vi "network_test_usrp.vi"() -> ()   [LabVIEW 2021]
uses:
  FPGA/reciver params.ctl
  Host/SubVIs/Start Trigger.ctl
  <instrlib>/niUsrpRio/Config/v1/Host/Public/niUsrpRio Session.ctl
  <instrlib>/_niInstr/Register Bus/v0/Host/Public/Register Bus Session.ctl
  <instrlib>/_niInstr/Register Bus/v0/Host/Private/Session Data.ctl
  <instrlib>/niUsrpRio/Config/v1/Host/Private/DB Queue Reference.ctl
  <instrlib>/niUsrpRio/Config/v1/Host/Private/Daughterboard Data.ctl
  <instrlib>/niUsrpRio/Config/v1/Host/Private/ATR state data.ctl
  <instrlib>/niUsrpRio/Config/v1/Host/Private/Antenna Configuration.ctl
  <instrlib>/niUsrpRio/Config/v1/Host/Private/CPLD Power Mode.ctl
  <instrlib>/niUsrpRio/Config/v1/Host/Public/EEPROM Header.ctl
  <instrlib>/niUsrpRio/Config/v1/Host/Public/EEPROM Device Data Header.ctl
  <instrlib>/niUsrpRio/Config/v1/Host/Public/EEPROM Characterization Header.ctl
  <instrlib>/niUsrpRio/Config/v1/Host/Public/Characterization Data.ctl
  <instrlib>/niUsrpRio/Config/v1/Host/Public/IQ Imbalance.ctl
  Host/SubVIs/Streaming Xvcr FPGA Ref.ctl
  <vilib>/userDefined/Silver/nirio_resource_slv.ctl
  Host/SubVIs/Initiate and Fetch (Multi).vi
  Host/SubVIs/Initiate and Fetch Time (Multi).vi
  <vilib>/Utility/error.llb/Error Cluster From Error Code.vi
  <vilib>/rvi/errors/niLvFpgaAdjustHostInterfaceError.vi
  Host/SubVIs/Initiate and Trigger.vi
  Host/SubVIs/Fetch Rx Data.vi
  Host/SubVIs/Fetch Rx Data (CDB WDT).vi
  Host/SubVIs/Check Aurora Link.vi
  Host/SubVIs/Check Stream Status.vi
  <vilib>/rvi/interface/nirviReadWriteControl/nirviReadWriteControl.xnode
  <vilib>/rvi/interface/nirviMethod/nirviMethod.xnode
  NiFpgaLv.dll
  <vilib>/rvi/interface/Simulation/niFpgaSimulationCallBeginRW.vi
  <vilib>/FPGAPlugInAG/Dynamic/niLvFpga_ReadFifo_Dynamic.vi
  <vilib>/rvi/errors/niLvFpgaMergeErrorWithErrorCode.vi
  <instrlib>/_niInstr/Register Bus/v0/Host/niInstr Register Bus v0 Host.lvlib
  <instrlib>/niUsrpRio/Config/v1/Host/niUsrpRio Config v1 Host.lvlib
  <vilib>/FPGAPlugInAG/Dynamic/niLvFpga_StopFifo_Dynamic.vi
  <vilib>/FPGAPlugInAG/Dynamic/niLvFpga_StartFifo_Dynamic.vi
panel:
  out "Ip - controler":string
  out "oders obay":dbl
  out "error out":errorcluster
  out "packege sent":u64
  out "state":T1(ring)
  out "data out 2":string
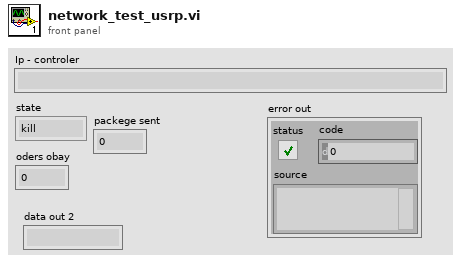
[diagram p1: front panel]
types:
  T1 = enum16{"kill", "turn off", "wait", "run", "turn on"}
  T2 = typedef "reciver params.ctl" = cluster{"min PW (fft cycels)":u16, "max PW (fft cycels)":u16, "max gap (fft cycels)":u8, "detection bar (liniar amp)":fxp<+,64,63>, "peak detect":bool}
  T3 = typedef "Start Trigger.ctl" = enum8{"Software", "Digital Edge", "Rx Start Trigger", "Tx Start Trigger", "Immediate", "Future Time Event"}
  T4 = typedef "niUsrpRio Config v1 Host.lvlib/niUsrpRio Session.ctl" = cluster{"FPGA Interface":refnum<k20>, "RIO Interface Number":u32, "Data Clock Rate":u32, "FPGA Data Clock Rate":u32, "Global Settings Register Bus":T5, "Radio 0 Settings Register Bus":T5, "Radio 1 Settings Register Bus":T5, "Radio Settings Bus Semaphore":T6, "DB Queues":T7[], "Characterization Data Valid?":bool, "EEPROM Header":T8, "Device Data Header":T9, "EEPROM Characterization Header":T10, "Characterization Data":T11[], "FPGA Current Version":u32, "FPGA Oldest Compatible Version":u32, "Fixed Logic Current Version":u32, "Fixed Logic Oldest Compatible Version":u32, "FPGA Radio Settings Bus Current Version":u32, "FPGA Radio Settings Bus Oldest Compatible Version":u32, "FPGA Board Config Current Version":u32, "FPGA Board Config Oldest Compatible Version":u32, "Daughterboard Clock Rate":u32, "daughterboard configuration session handles":u64[]}
  T5 = typedef "niInstr Register Bus v0 Host.lvlib/Register Bus Session.ctl" = refnum<queue>
  T6 = typedef "Semaphore RefNum" = refnum<k1>
  T7 = typedef "niUsrpRio Config v1 Host.lvlib/DB Queue Reference.ctl" = refnum<queue>
  T8 = typedef "niUsrpRio Config v1 Host.lvlib/EEPROM Header.ctl" = cluster{"Checksum":u32, "Product Code":u16, "Hardware Current Version":u16, "Hardware Oldest Compatible Version":u16, "EEPROM Map Current Version":u16, "EEPROM Map Oldest Compatible Version":u16, "User Password":string, "Pointer to Factory Header":u32, "Pointer to User Header":u32, "Recommended Interval":u16, "Number of Reserved Bytes":i32, "Number of Daughterboards":u8, "Daughterboard IDs":u16[], "Daughterboard Serial Numbers":string[]}
  T9 = typedef "niUsrpRio Config v1 Host.lvlib/EEPROM Device Data Header.ctl" = cluster{"Checksum":u32, "Number of Channels":u8, "Number of Gain Settings":u16[], "Pointer to Characterization Data":u32[], "Number of Reserved Bytes":i32, "Number of Frequencies":u16[]}
  T10 = typedef "niUsrpRio Config v1 Host.lvlib/EEPROM Characterization Header.ctl" = cluster{"Checksum":u32, "Date":timestamp, "Temperature":sgl, "Misc. Info":string, "Pointer to Device Data Header":u32, "Number of Reserved Bytes":i32}
  T11 = typedef "niUsrpRio Config v1 Host.lvlib/Characterization Data.ctl" = cluster{"Gains[dB]":dbl[], "Frequencies [Hz]":dbl[], "IQ Imbalance Table":T12[], "Measured Gains[dB]":dbl[][]}
  T12 = typedef "niUsrpRio Config v1 Host.lvlib/IQ Imbalance.ctl" = cluster{"Gain Imbalance [linear]":dbl, "Phase Imbalance [radians]":dbl, "Offset":cdb}
  T13 = cluster{"state":enum16{"kill", "turn off", "wait", "run", "turn on"}, "queue out":refnum<queue>, "reciver_params":T2, "port":refnum<k16>, "rx config":cluster{"rf enable 0":bool, "rf config 0":cluster{"antenna":string, "frequency":dbl, "lo frequency":dbl, "level":dbl}, "rf enable 1":bool, "rf config 1":cluster{"antenna":string, "frequency":dbl, "lo frequency":dbl, "level":dbl}, "transfer mode":enum16{"Finite", "Continuous"}, "sample rate":dbl, "number of samples":u32, "start trigger":T3}, "niUsrpRio Session (out)":T4}
  T14 = cluster{"rf enable 0":bool, "rf config 0":cluster{"antenna":string, "frequency":dbl, "lo frequency":dbl, "level":dbl}, "rf enable 1":bool, "rf config 1":cluster{"antenna":string, "frequency":dbl, "lo frequency":dbl, "level":dbl}, "transfer mode":enum16{"Finite", "Continuous"}, "sample rate":dbl, "number of samples":u32, "start trigger":T3}
  T15 = typedef "Streaming Xvcr FPGA Ref.ctl" = refnum<k20>
  T16 = typedef "nirio_resource_slv.ctl" = tag
  T17 = cluster{"rx.state":enum16{"Idle", "Active"}, "rx.samples processed":u32, "rx.number of fifo overflows":u32, "rx.number of iq data overflows":u64[], "rx.dsp reset done":bool}
  T18 = typedef "Rx Channels.ctl" = cluster{"rx config":cluster{"channel configuration":cluster{"channel enable":bool, "channel configuration":cluster{"antenna":string, "frequency":dbl, "lo frequency":dbl, "level":dbl}}[], "transfer mode":enum16{"Finite", "Continuous"}, "sample rate":dbl, "number of samples":u32, "start trigger":T3}, "reference frequency source":string, "rx.data sink":enum16{"SFP Port 0", "SFP Port 1", "Host"}, "rx.enabled channels":string[], "vertical range":dbl[], "rx.coerced configurations":cluster{"coerced frequencies":dbl[], "coerced lo frequencies":dbl[], "coerced levels":dbl[], "coerced sample rates":dbl[]}}
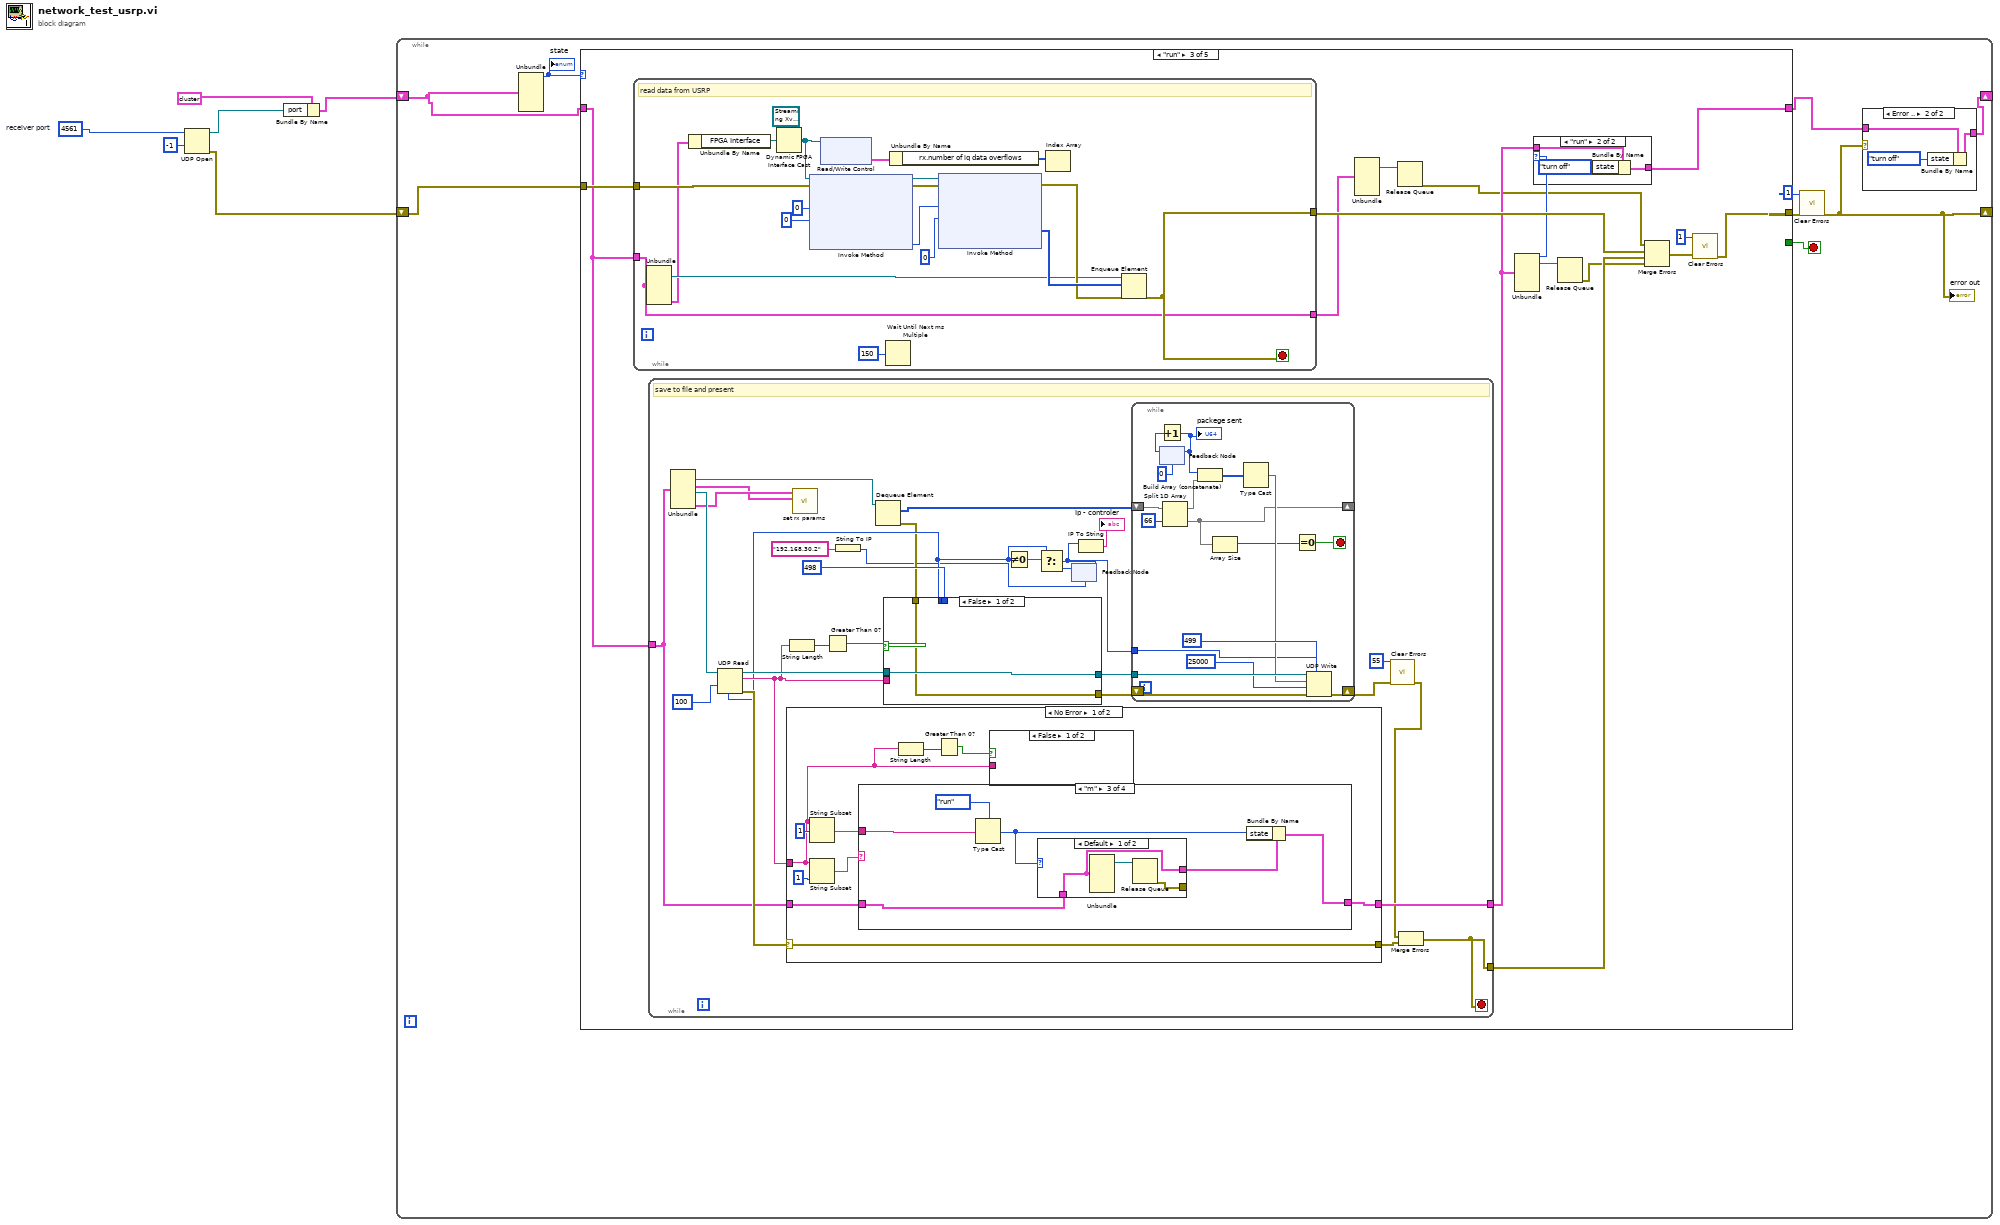
[diagram p0: block diagram]
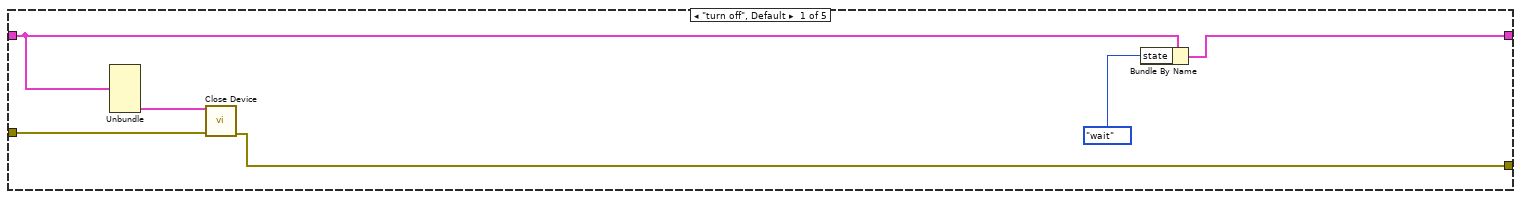
[diagram p3: hidden frame]
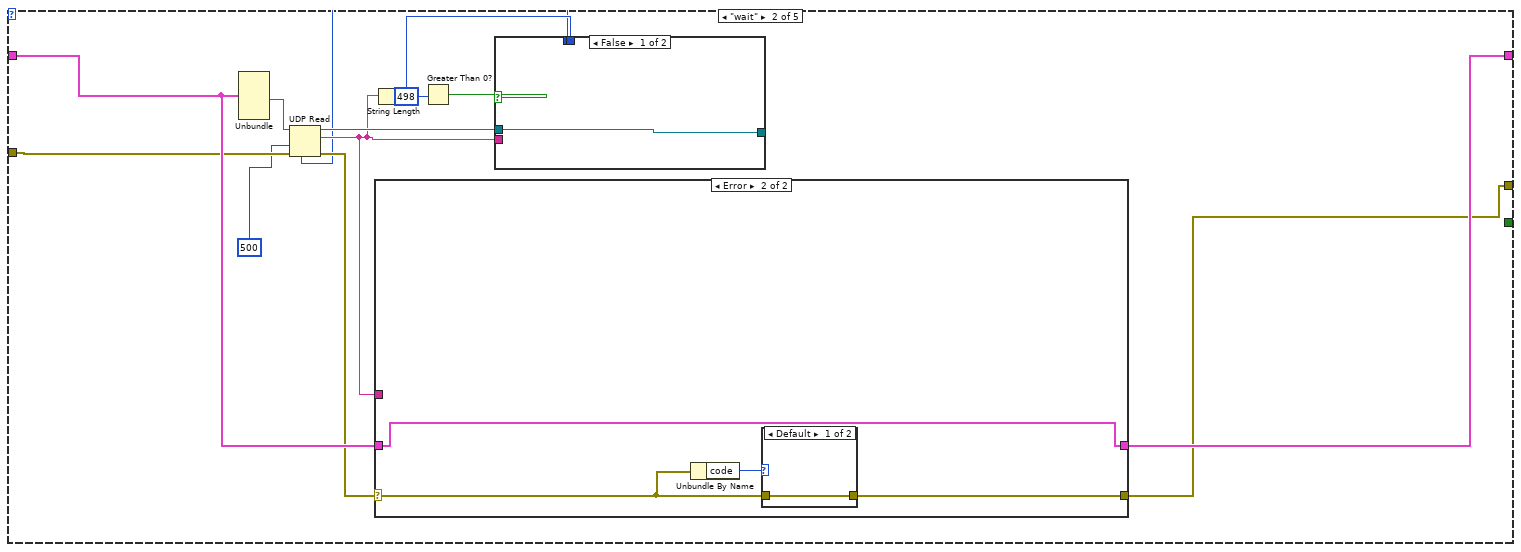
[diagram p4: hidden frame]
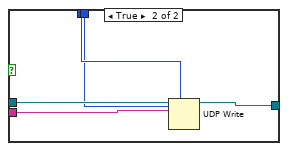
[diagram p5: hidden frame]
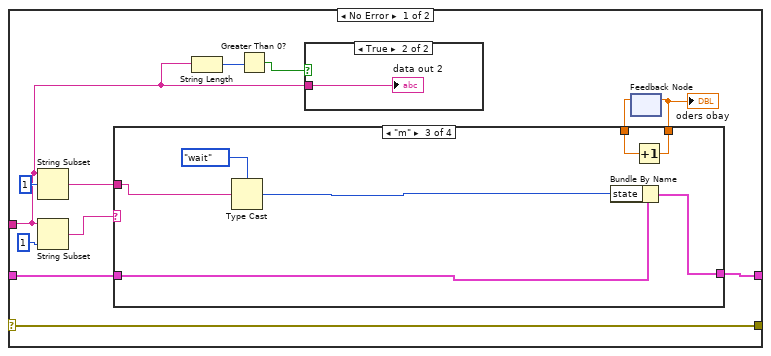
[diagram p6: hidden frame]
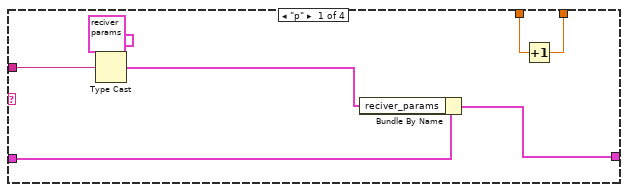
[diagram p8: hidden frame]
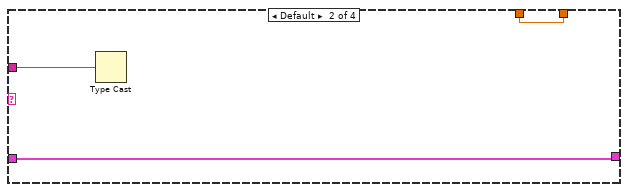
[diagram p9: hidden frame]
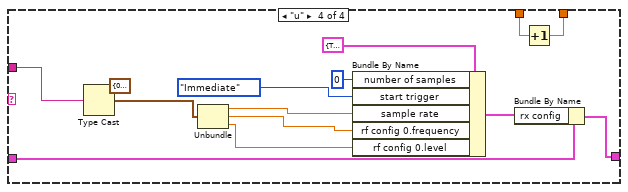
[diagram p10: hidden frame]
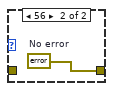
[diagram p11: hidden frame]
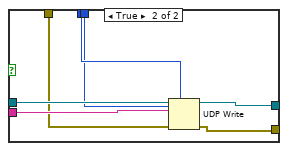
[diagram p13: hidden frame]
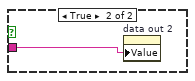
[diagram p14: hidden frame]
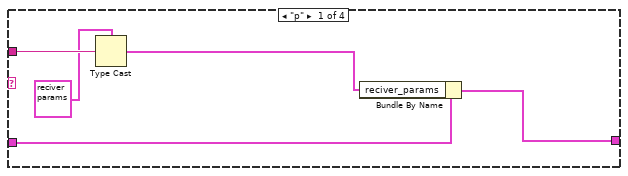
[diagram p15: hidden frame]
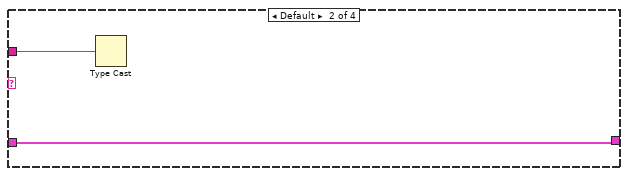
[diagram p16: hidden frame]
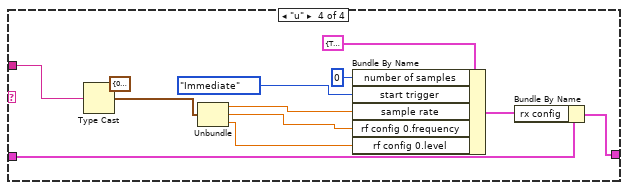
[diagram p18: hidden frame]
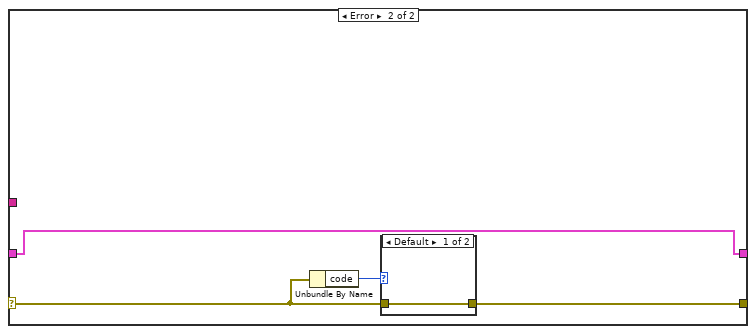
[diagram p19: hidden frame]
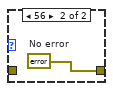
[diagram p20: hidden frame]
diagram:
  w6 = u16 4561  # receiver port
  n1 = UDP Open(9:-1 ("timeout ms (25000)"), 11:w6) -> (port=w3:refnum<k16>, 0:w2:errorcluster)  [unwired: 3 in, 1 out]
  n2 = Bundle By Name(cluster=T13 {"state"=enum."wait", "queue out"=refnum, "reciver_params"={"min PW (fft cycels)"=0, "max PW (fft cycels)"=1500, "max gap (fft cycels)"=0, "detection bar (liniar amp)"=93.0, "peak detect"=FALSE}, "port"=refnum, "rx config"={"rf enable 0"=TRUE, "rf config 0"={"antenna"="RX1", "frequency"=2000000000.0, "lo frequency"=-1.0, "level"=0.0}, "rf enable 1"=FALSE, "rf config 1"={"antenna"="RX2", "frequency"=2000000000.0, "lo frequency"=-1.0, "level"=0.0}, "transfer mode"=enum."Continuous", "sample rate"=10000000.0, "number of samples"=4194304, "start trigger"=enum."Immediate"}, "niUsrpRio Session (out)"={"FPGA Interface"=refnum, "RIO Interface Number"=0, "Data Clock Rate"=0, "FPGA Data Clock Rate"=0, "Global Settings Register Bus"=refnum, "Radio 0 Settings Register Bus"=refnum, "Radio 1 Settings Register Bus"=refnum, "Radio Settings Bus Semaphore"=refnum, "DB Queues"=[], "Characterization Data Valid?"=FALSE, "EEPROM Header"={"Checksum"=0, "Product Code"=0, "Hardware Current Version"=0, "Hardware Oldest Compatible Version"=0, "EEPROM Map Current Version"=0, "EEPROM Map Oldest Compatible Version"=0, "User Password"="", "Pointer to Factory Header"=0, "Pointer to User Header"=0, "Recommended Interval"=0, "Number of Reserved Bytes"=9, "Number of Daughterboards"=0, "Daughterboard IDs"=[], "Daughterboard Serial Numbers"=[]}, "Device Data Header"={"Checksum"=0, "Number of Channels"=0, "Number of Gain Settings"=[], "Pointer to Characterization Data"=[], "Number of Reserved Bytes"=27, "Number of Frequencies"=[]}, "EEPROM Characterization Header"={"Checksum"=0, "Date"=timestamp(0 s since 1904-01-01), "Temperature"=0.0, "Misc. Info"="", "Pointer to Device Data Header"=0, "Number of Reserved Bytes"=28}, "Characterization Data"=[], "FPGA Current Version"=0, "FPGA Oldest Compatible Version"=0, "Fixed Logic Current Version"=0, "Fixed Logic Oldest Compatible Version"=0, "FPGA Radio Settings Bus Current Version"=0, "FPGA Radio Settings Bus Oldest Compatible Version"=0, "FPGA Board Config Current Version"=0, "FPGA Board Config Oldest Compatible Version"=0, "Daughterboard Clock Rate"=0, "daughterboard configuration session handles"=[]}}, "port"=w3) -> (w1:T13)
  n3 = while {
    shift-right: [w7] -> _
    shift-left: w2 -> [w14]
    shift-right: [w8] -> _
    shift-left: w1 -> [w12]
    stop <- w15 stop-if-true
    n4 = Unbundle(w12) -> ("state"=w13:T1)  [unwired: 5 out]
    "state" <- w13
    n5 = case shown="\"run\"" w13 {
      tunnel: [_ _ _ _ TRUE] -> w15
      tunnel: [w20 w26 w104 w246 _] -> w10
      tunnel: w14 -> [w21 w36 w109 _ _]
      tunnel: [w23 w37 w98 w243 w258] -> w9
      tunnel: w12 -> [w24 w38 w108 w244 w258]
      frame "turn off", Default {
        n6 = Unbundle(w24) -> ("niUsrpRio Session (out)"=w25:T4)  [unwired: 5 out]
        n7 = call "Close Device.vi"("niUsrpRio Session"=w25, "error in"=w21) -> ("error out"=w20:errorcluster)  [unwired: 13 in]
        n8 = Bundle By Name(cluster=w24, "state"=T1."wait") -> (w23:T13)
      }
      frame "wait" {
        n9 = Unbundle(w38) -> ("port"=w29:refnum<k16>)  [unwired: 5 out]
        n10 = UDP Read(connection ID=w29, timeout ms (25000)=500, 8:w36) -> (data out=w31:string, error out=w35:errorcluster, 3:w34:refnum<k16>, 6:w28:u32)  [unwired: 2 out]
        n11 = case shown="Error" w35 {
          selector: w35 -> [w56 w91]
          tunnel: [w56 w90] -> w26
          tunnel: w31 -> [w49 _]
          tunnel: w38 -> [w51 w89]
          tunnel: [w50 w89] -> w37
          frame No Error {
            # "Sender sent data. Update the chart value."
            n12 = String Subset(string=w49, offset (0)=1) -> (substring=w53:string)  [unwired: 1 in]
            n13 = String Subset(string=w49, length (rest)=1 ("length (rest)")) -> (substring=w52:string)  [unwired: 1 in]
            n14 = String Length(string=w49) -> (length=w48:i32)
            n15 = Greater Than 0?(x=w48) -> (x > 0?=w47:bool)
            n16 = case shown="True" w47 {
              tunnel: w49 -> [_ w57]
              frame False {
              }
              frame True {
                "data out 2" <- w57
              }
            }
            n17 = feedback #1() -> (w45:dbl)  [unwired: 1 in]
            n18 = case shown="\"m\"" w52 {
              tunnel: w53 -> [w64 w67 w74 w88]
              tunnel: w51 -> [w62 w66 w72 w86]
              tunnel: [w61 w66 w71 w85] -> w50
              tunnel: [w59 w65 w68 w75] -> w46
              tunnel: w45 -> [w58 w65 w69 w76]
              frame "p" {
                n19 = Type Cast(type=T2 {"min PW (fft cycels)"=5, "max PW (fft cycels)"=500, "max gap (fft cycels)"=1, "detection bar (liniar amp)"=1000000.0, "peak detect"=FALSE} ("reciver_params"), x=w64) -> (*(type *) &x=w60:T2)
                n20 = Bundle By Name(cluster=w62, "reciver_params"=w60) -> (w61:T13)
                n21 = Increment(x=w58) -> (x+1=w59:dbl)
              }
              frame Default {
                n22 = Type Cast(x=w67) -> ()  [unwired: 1 in, 1 out]
              }
              frame "m" {
                n23 = Type Cast(type=T1."wait", x=w74) -> (*(type *) &x=w70:T1)
                n24 = Bundle By Name(cluster=w72, "state"=w70) -> (w71:T13)
                n25 = Increment(x=w69) -> (x+1=w68:dbl)
              }
              frame "u" {
                n26 = Type Cast(type=cluster{dbl, dbl, dbl} {0.0, 0.0, 0.0}, x=w88) -> (*(type *) &x=w84:cluster{dbl, dbl, dbl})
                n27 = Unbundle(w84) -> (w80:dbl, w78:dbl, w79:dbl)
                n28 = Bundle By Name(cluster=T14 {"rf enable 0"=TRUE, "rf config 0"={"antenna"="RX1", "frequency"=2000000000.0, "lo frequency"=-1.0, "level"=0.0}, "rf enable 1"=FALSE, "rf config 1"={"antenna"="RX2", "frequency"=2000000000.0, "lo frequency"=-1.0, "level"=0.0}, "transfer mode"=enum."Continuous", "sample rate"=10000000.0, "number of samples"=4194304, "start trigger"=enum."Immediate"} ("rx config"), "number of samples"=u32 0, "start trigger"=Start_Trigger."Immediate", "sample rate"=w80, "rf config 0.frequency"=w78, "rf config 0.level"=w79) -> (w82:T14)
                n29 = Bundle By Name(cluster=w86, "rx config"=w82) -> (w85:T13)
                n30 = Increment(x=w76) -> (x+1=w75:dbl)
              }
            }
            "oders obay" <- w46
            n31 = feedback-in #1(w46) -> ()
          }
          frame Error {
            # "Sender did not send data. Ignore timeout error and keep waiting."
            n32 = Unbundle By Name(w91) -> ("code"=w92:i32)
            n33 = case shown="Default" w92 {
              tunnel: w91 -> [w93 _]
              tunnel: [w93 w94] -> w90
              frame Default {
              }
              frame 56 {
                w94 = errorcluster {"status"=FALSE, "code"=0, "source"=""}  # No error
              }
            }
          }
        }
        n34 = String Length(string=w31) -> (length=w32:i32)
        n35 = Greater Than 0?(x=w32) -> (x > 0?=w30:bool)
        n36 = case shown="False" w30 {
          tunnel: w34 -> [w39 w44]
          tunnel: [w39 w43] -> _
          tunnel: w28 -> [_ w42]
          tunnel: u16 498 ("port or service name") -> [_ w41]
          tunnel: w31 -> [_ w40]
          frame False {
          }
          frame True {
            n37 = UDP Write(address=w42, port or service name=w41, connection ID=w44, data in=w40) -> (3:w43:refnum<k16>)  [unwired: 2 in, 1 out]
          }
        }
      }
      frame "run" {
        n38 = while {
          tunnel: [w216] -> w106
          tunnel: w109 -> [w222]
          tunnel: w108 -> [w215]
          tunnel: [w215] -> w96
          stop <- w216 stop-if-true
          # "read data from USRP"
          n39 = Unbundle(w215) -> ("queue out"=w218:refnum<queue>, "niUsrpRio Session (out)"=w217:T4)  [unwired: 4 out]
          n40 = Unbundle By Name(w217) -> ("FPGA Interface"=w233:refnum<k20>)
          n41 = Dynamic FPGA Interface Cast(Session In=T15 refnum ("Type"), Type=w233) -> (Session Out=w224:T15)
          n42 = xnode "Invoke Method"("FPGA VI Reference In"=w224, "error in"=w222, "Number of Elements"=u32 0, "Timeout (ms)"=0) -> ("FPGA VI Reference Out"=w220:T15, "error out"=w223:errorcluster, "Elements Remaining"=w229:u32)  [unwired: 1 out]
          n43 = xnode "Read/Write Control"("FPGA VI Reference In"=w224) -> ("rx.status"=w231:T17)  [unwired: 1 in, 2 out]
          n44 = Wait Until Next ms Multiple(millisecond multiple=u32 150) -> ()  [unwired: 1 out]
          n45 = Unbundle By Name(w231) -> ("rx.number of iq data overflows"=w230:u64[])
          n46 = xnode "Invoke Method"("FPGA VI Reference In"=w220, "error in"=w223, "Number of Elements"=w229, "Timeout (ms)"=0) -> ("error out"=w221:errorcluster, "Data"=w226:u64[])  [unwired: 2 out]
          n47 = Index Array(array=w230) -> ()  [unwired: 1 in, 1 out]
          n48 = Enqueue Element(queue=w218, element=w226, error in (no error)=w221) -> (error out=w216:errorcluster)  [unwired: 1 in, 2 out]
        }
        n49 = while {
          tunnel: w108 -> [w135]
          tunnel: [w134] -> w99
          tunnel: [w123] -> w107
          stop <- w123 stop-if-true
          # "save to file and present"
          n50 = Unbundle(w135) -> ("queue out"=w130:refnum<queue>, "reciver_params"=w131:T2, "port"=w133:refnum<k16>, "niUsrpRio Session (out)"=w132:T4)  [unwired: 2 out]
          n51 = UDP Read(connection ID=w133, timeout ms (25000)=100) -> (data out=w137:string, error out=w141:errorcluster, 3:w140:refnum<k16>, 6:w126:u32)  [unwired: 1 in, 2 out]
          n52 = case shown="No Error" w141 {
            selector: w141 -> [w178 w211]
            tunnel: [w178 w210] -> w124
            tunnel: w137 -> [w169 _]
            tunnel: w135 -> [w173 w209]
            tunnel: [w172 w209] -> w134
            frame No Error {
              # "Sender sent data. Update the chart value."
              n53 = String Subset(string=w169, offset (0)=1) -> (substring=w175:string)  [unwired: 1 in]
              n54 = String Subset(string=w169, length (rest)=1 ("length (rest)")) -> (substring=w174:string)  [unwired: 1 in]
              n55 = case shown="\"m\"" w174 {
                tunnel: w175 -> [w184 w186 w192 w208]
                tunnel: w173 -> [w182 w185 w188 w206]
                tunnel: [w181 w185 w190 w205] -> w172
                frame "p" {
                  n56 = Type Cast(type=T2 {"min PW (fft cycels)"=5, "max PW (fft cycels)"=500, "max gap (fft cycels)"=1, "detection bar (liniar amp)"=1000000.0, "peak detect"=FALSE} ("reciver_params"), x=w184) -> (*(type *) &x=w180:T2)
                  n57 = Bundle By Name(cluster=w182, "reciver_params"=w180) -> (w181:T13)
                }
                frame Default {
                  n58 = Type Cast(x=w186) -> ()  [unwired: 1 in, 1 out]
                }
                frame "m" {
                  n59 = Type Cast(type=T1."run", x=w192) -> (*(type *) &x=w189:T1)
                  n60 = case shown="Default" w189 {
                    tunnel: [w194 w196] -> w187
                    tunnel: w188 -> [w194 w196]
                    tunnel: [w193 _] -> _
                    frame Default {
                      n61 = Unbundle(w194) -> ("queue out"=w195:refnum<queue>)  [unwired: 5 out]
                      n62 = Release Queue(queue=w195) -> (error out=w193:errorcluster)  [unwired: 2 in, 2 out]
                    }
                    frame "run" {
                    }
                  }
                  n63 = Bundle By Name(cluster=w187, "state"=w189) -> (w190:T13)
                }
                frame "u" {
                  n64 = Type Cast(type=cluster{dbl, dbl, dbl} {0.0, 0.0, 0.0}, x=w208) -> (*(type *) &x=w204:cluster{dbl, dbl, dbl})
                  n65 = Unbundle(w204) -> (w200:dbl, w198:dbl, w199:dbl)
                  n66 = Bundle By Name(cluster=T14 {"rf enable 0"=TRUE, "rf config 0"={"antenna"="RX1", "frequency"=2000000000.0, "lo frequency"=-1.0, "level"=0.0}, "rf enable 1"=FALSE, "rf config 1"={"antenna"="RX2", "frequency"=2000000000.0, "lo frequency"=-1.0, "level"=0.0}, "transfer mode"=enum."Continuous", "sample rate"=10000000.0, "number of samples"=4194304, "start trigger"=enum."Immediate"} ("rx config"), "number of samples"=u32 0, "start trigger"=Start_Trigger."Immediate", "sample rate"=w200, "rf config 0.frequency"=w198, "rf config 0.level"=w199) -> (w202:T14)
                  n67 = Bundle By Name(cluster=w206, "rx config"=w202) -> (w205:T13)
                }
              }
              n68 = String Length(string=w169) -> (length=w171:i32)
              n69 = Greater Than 0?(x=w171) -> (x > 0?=w170:bool)
              n70 = case shown="False" w170 {
                tunnel: w169 -> [_ w179]
                frame False {
                }
                frame True {
                  n71 = property on="data out 2" class="Str"("Value"=w179) -> ()  [unwired: 2 in, 2 out]
                }
              }
            }
            frame Error {
              # "Sender did not send data. Ignore timeout error and keep waiting."
              n72 = Unbundle By Name(w211) -> ("code"=w212:i32)
              n73 = case shown="Default" w212 {
                tunnel: w211 -> [w213 _]
                tunnel: [w213 w214] -> w210
                frame Default {
                }
                frame 56 {
                  w214 = errorcluster {"status"=FALSE, "code"=0, "source"=""}  # No error
                }
              }
            }
          }
          n74 = String Length(string=w137) -> (length=w138:i32)
          n75 = call "set rx params.vi"("reciver_params"=w131, "niUsrpRio Session (out)"=w132) -> ()  [unwired: 8 in, 2 out]
          n76 = Greater Than 0?(x=w138) -> (x > 0?=w136:bool)
          n77 = String To IP(1:"192.168.30.2" ("name")) -> (0:w120:u32)
          n78 = Dequeue Element(queue=w130) -> (element=w119:u64[], error out=w122:errorcluster)  [unwired: 2 in, 2 out]
          n79 = case shown="False" w136 {
            tunnel: w140 -> [w161 w168]
            tunnel: [w161 w167] -> w129
            tunnel: w126 -> [_ w166]
            tunnel: u16 498 ("port or service name") -> [_ w165]
            tunnel: w137 -> [_ w164]
            tunnel: [w160 w163] -> w128
            tunnel: w122 -> [w160 w162]
            frame False {
            }
            frame True {
              n80 = UDP Write(address=w166, port or service name=w165, connection ID=w168, data in=w164, 8:w162) -> (error out=w163:errorcluster, 3:w167:refnum<k16>)  [unwired: 1 in]
            }
          }
          n81 = Not Equal To 0?(x=w126) -> (x != 0?=w127:bool)
          n82 = feedback #2(w120) -> (w125:u32)
          n83 = Select(t=w126, s=w127, f=w125) -> (s? t:f=w115:u32)
          n84 = feedback-in #2(w115) -> ()
          n85 = IP To String(2:w115) -> (0:→"Ip - controler":string)  [unwired: 1 in]
          n86 = while {
            tunnel: w129 -> [w159]
            tunnel: w115 -> [w153]
            shift-right: [w152] -> w118
            shift-left: w128 -> [w155]
            shift-right: [w146] -> _
            shift-left: w119 -> [w150]
            stop <- w145 stop-if-true
            n87 = feedback #3(u64 0) -> (w156:u64)
            n88 = Increment(x=w156) -> (x+1=w149:u64)
            "packege sent" <- w149
            n89 = feedback-in #3(w149) -> ()
            n90 = Split 1D Array(array=w150, index=66) -> (first subarray=w148:u64[], second subarray=w146:u64[])
            n91 = Build Array (concatenate)(w149, w148) -> (w147:u64[])
            n92 = Array Size(array=w146) -> (size(s)=w144:i32)
            n93 = Type Cast(x=w147) -> (*(type *) &x=w157:string)  [unwired: 1 in]
            n94 = Equal To 0?(x=w144) -> (x = 0?=w145:bool)
            n95 = UDP Write(address=w153, port or service name=u16 499, connection ID=w159, data in=w157, 8:w155, 9:25000 ("timeout ms (25000)")) -> (error out=w152:errorcluster)  [unwired: 1 out]
          }
          n96 = call <vilib>:"Clear Errors.vi"("error in (no error)"=w118, "specific error code to clear (0: all)"=55) -> ("error out"=w117:errorcluster)  [unwired: 4 in, 1 out]
          n97 = Merge Errors(w117, w124) -> (w123:errorcluster)
        }
        n98 = Unbundle(w96) -> ("queue out"=w97:refnum<queue>)  [unwired: 5 out]
        n99 = Release Queue(queue=w97) -> (error out=w95:errorcluster)  [unwired: 2 in, 2 out]
        n100 = Unbundle(w99) -> ("state"=w100:T1, "queue out"=w102:refnum<queue>)  [unwired: 4 out]
        n101 = case shown="\"run\"" w100 {
          tunnel: w99 -> [w110 w113]
          tunnel: [w110 w111] -> w98
          frame "kill", Default {
          }
          frame "run" {
            n102 = Bundle By Name(cluster=w113, "state"=T1."turn off") -> (w111:T13)
          }
        }
        n103 = Release Queue(queue=w102) -> (error out=w101:errorcluster)  [unwired: 2 in, 2 out]
        n104 = Merge Errors(w95, w106, w107, w101) -> (w105:errorcluster)
        n105 = call <vilib>:"Clear Errors.vi"("error in (no error)"=w105, "specific error code to clear (0: all)"=1) -> ("error out"=w104:errorcluster)  [unwired: 4 in, 1 out]
      }
      frame "turn on" {
        n106 = Unbundle(w244) -> ("rx config"=w245:T14)  [unwired: 5 out]
        n107 = call "Open and Configure Device.vi"("USRP RIO Device"=T16 "RIO0" ("USRP RIO device"), "reference frequency source"="Internal", "which bitfile"="Time", "rx config"=w245) -> ("rx channels"=w254:T18, "niUsrpRio Session (out)"=w251:T4, "error out"=w252:errorcluster)  [unwired: 5 in, 4 out]
        n108 = call "Initiate and Fetch (Single).vi"("niUsrpRio Session"=w251, "rx channels"=w254, "first iteration"=TRUE, "error in"=w252) -> ("niUsrpRio Session (out)"=w237:T4, "error out"=w247:errorcluster)  [unwired: 9 in, 1 out]
        n109 = Obtain Queue(max queue size (-1, unlimited)=100000000, element data type=u64[] [] ("waveform data")) -> (queue out=w241:refnum<queue>, error out=w248:errorcluster)  [unwired: 3 in, 1 out]
        n110 = Unbundle By Name(w237) -> ("FPGA Interface"=w240:refnum<k20>)
        n111 = Bundle By Name(cluster=w244, "state"=T1."run", "niUsrpRio Session (out)"=w237, "queue out"=w241) -> (w243:T13)
        n112 = Dynamic FPGA Interface Cast(Session In=T15 refnum ("Type"), Type=w240) -> (Session Out=w238:T15)
        n113 = xnode "Invoke Method"("FPGA VI Reference In"=w238) -> ("FPGA VI Reference Out"=w236:T15, "error out"=w235:errorcluster)  [unwired: 1 in]
        n114 = xnode "Invoke Method"("FPGA VI Reference In"=w236, "error in"=w235) -> ("error out"=w234:errorcluster)  [unwired: 1 out]
        n115 = Merge Errors(w248, w247, w234) -> (w246:errorcluster)
      }
      frame "kill" {
      }
    }
    n116 = call <vilib>:"Clear Errors.vi"("error in (no error)"=w10, "specific error code to clear (0: all)"=1) -> ("error out"=w7:errorcluster)  [unwired: 4 in, 1 out]
    "error out" <- w7
    n117 = case shown="Error .." w7 {
      tunnel: [w16 w18] -> w8
      tunnel: w9 -> [w16 w19]
      frame No Error {
      }
      frame Error {
        n118 = Bundle By Name(cluster=w19, "state"=T1."turn off") -> (w18:T13)
      }
    }
  }
